vi "系统设置.vi"() -> ()   [LabVIEW 2016]
uses:
  <vilib>/Utility/miscctls.llb/LVPointTypeDef.ctl
  <vilib>/Utility/config.llb/Read Key (U32).vi
  <vilib>/Utility/config.llb/Write Key (I32).vi
  <vilib>/ptbypt/NI_PtbyPt.lvlib
  PLC/PLC.lvlib
  <vilib>/Utility/config.llb/NI_LVConfig.lvlib
panel:
  in  "24H周期设置":T1(xcontrol)
  in  "采水模式":enum16{"使用采水泵", "不使用采水泵"}(ring)
  in  "运行模式":enum16{"维护模式", "常规模式", "应急模式", "质控模式"}(ring)
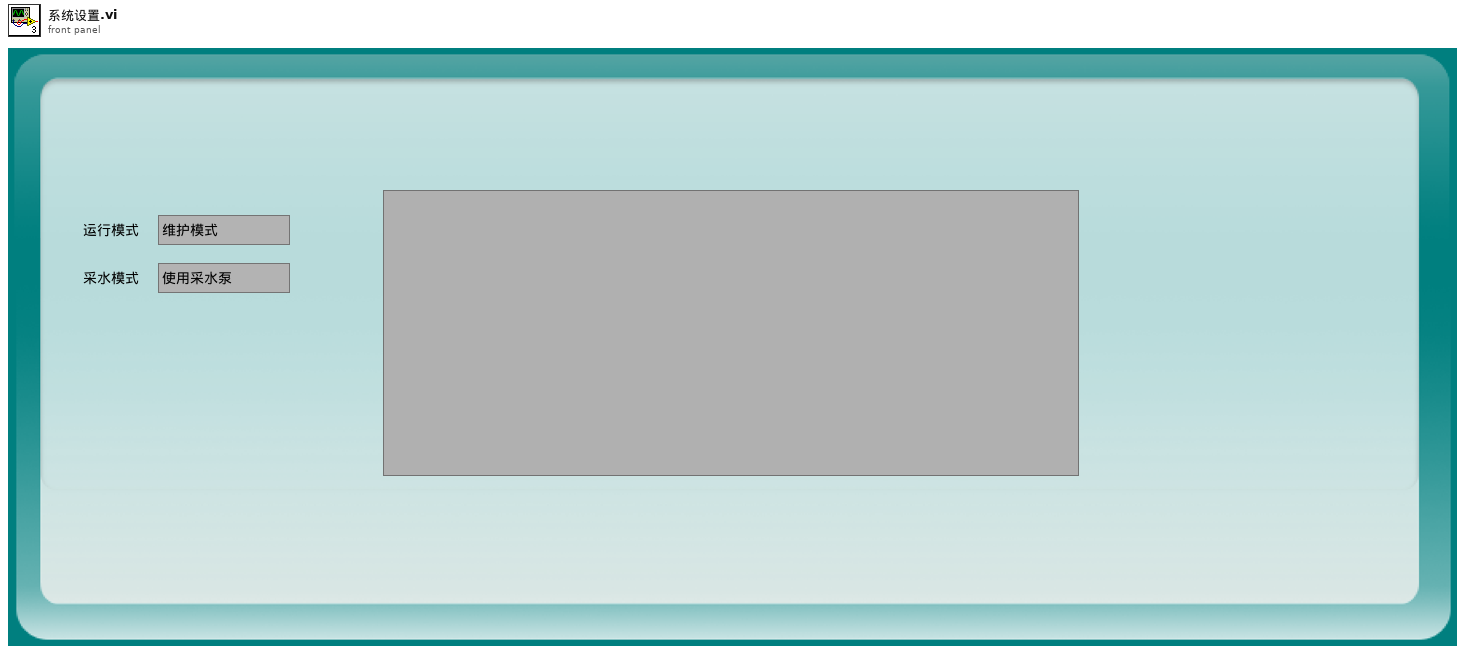
[diagram p1: front panel]
types:
  T1 = cluster{"00H":bool, "01H":bool, "02H":bool, "03H":bool, "04H":bool, "05H":bool, "06H":bool, "07H":bool, "08H":bool, "09H":bool, "10H":bool, "11H":bool, "12H":bool, "13H":bool, "14H":bool, "15H":bool, "16H":bool, "17H":bool, "18H":bool, "19H":bool, "20H":bool, "21H":bool, "22H":bool, "23H":bool}
  T2 = typedef "LVPointTypeDef.ctl" = cluster{"Horizontal":i16, "Vertical":i16}
  T3 = typedef "NI_LVConfig.lvlib/Config Data RefNum.ctl" = refnum<k1>
  T4 = cluster{"是否启用仪器":bool, "CODMn":cluster{"启动测量模式":cluster{"测量模式":enum16{"水样测量", "标样核查", "零点核查", "加标回收", "平行样", "校零", "校标"}}, "确定按钮":bool}, "采水模式":enum16{"使用采水泵", "不使用采水泵"}}
  T5 = enum16{"水样测量", "标样核查", "零点核查", "加标回收", "平行样", "校零", "校标"}
  T6 = cluster{"运行模式":enum16{"维护模式", "常规模式", "应急模式", "质控模式"}}
  T7 = typedef "LVDateTimeRec.ctl" = cluster{"秒数的小数部分":dbl, "秒":i32, "分":i32, "时":i32, "日":i32, "月":i32, "年":i32, "天数（周）":i32, "天数（年）":i32, "DST":i32}
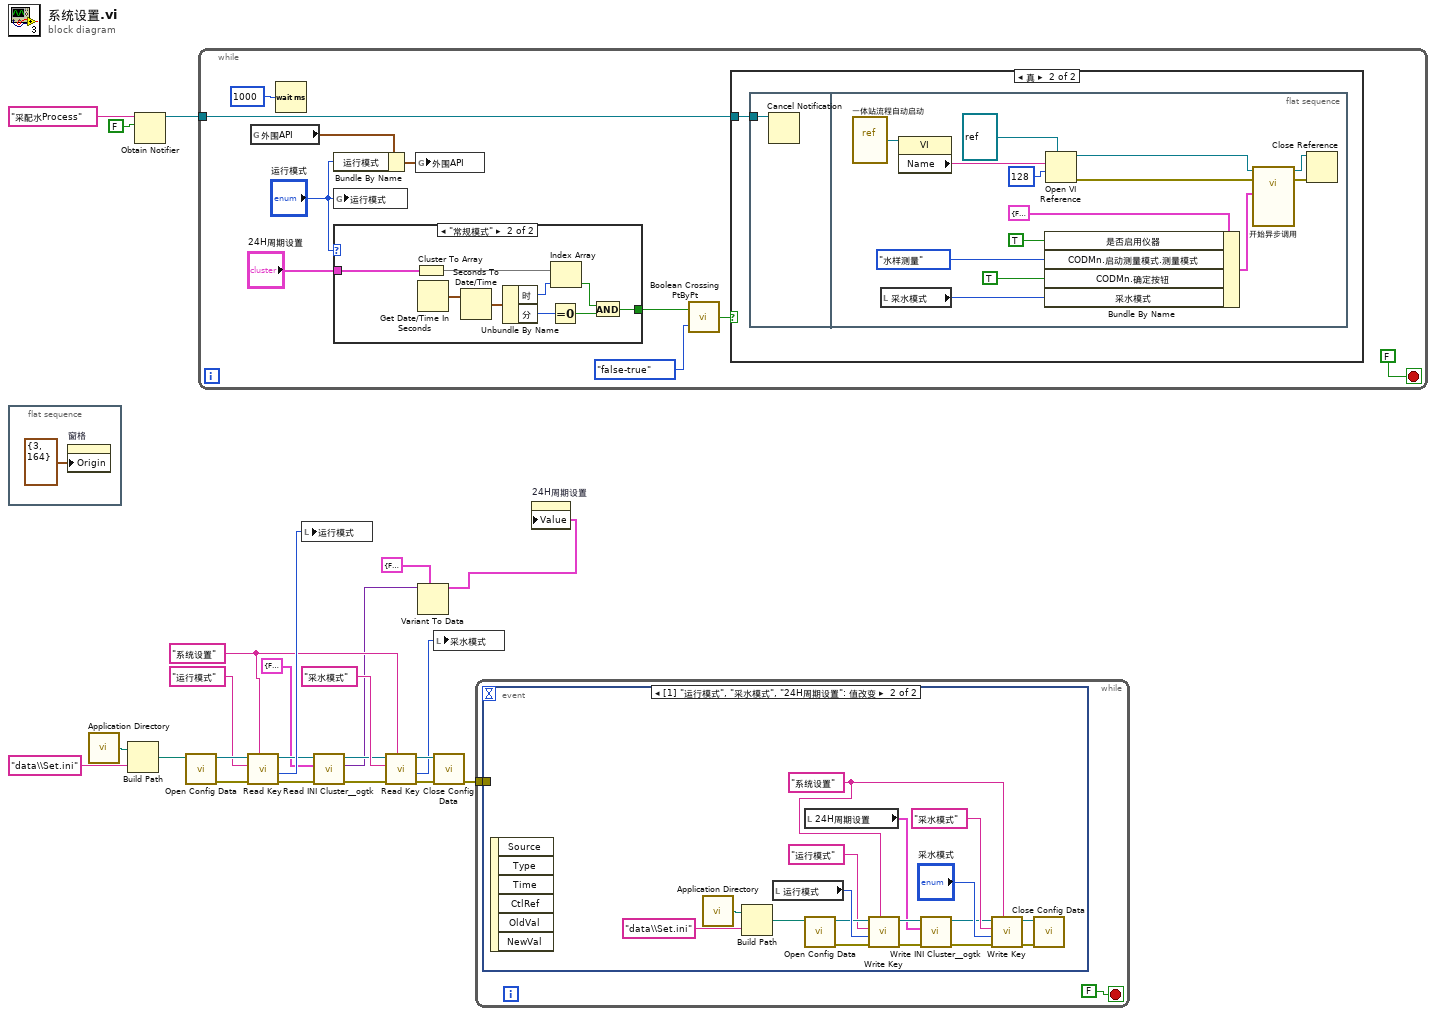
[diagram p0: block diagram]
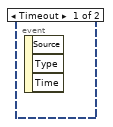
[diagram p4: hidden frame]
diagram:
  w9 = "系统设置" ("section")
  n1 = flat-sequence {
    frame #0 {
      n2 = property on="窗格" class="Pane"("Origin"=T2 {"Horizontal"=3, "Vertical"=164} ("原点")) -> ()  [unwired: 2 in, 2 out]
    }
  }
  n3 = call <vilib>:"Application Directory.vi"() -> ("Application Directory"=w19:path)
  n4 = Build Path(base path=w19, name or relative path="data\\Set.ini" ("名称或相对路径")) -> (appended path=w17:path)
  n5 = Obtain Notifier(name (unnamed)="采配水Process" ("名称（未命名）"), notification data type=FALSE) -> (notifier out=w22:refnum<notifier>)  [unwired: 2 in, 2 out]
  n6 = call <vilib>:"Open Config Data.vi"("configuration file path"=w17) -> ("error out"=w20:errorcluster, "refnum"=w21:T3)  [unwired: 8 in, 1 out]
  n7 = while {
    tunnel: w22 -> [w33]
    stop <- FALSE stop-if-true
    n8 = global read "VAR总磷氨氮全局变量.vi" "外围API"() -> (w28:T6)
    n9 = Wait (ms)(milliseconds to wait=u32 1000 ("等待时间（毫秒）")) -> ()  [unwired: 1 out]
    n10 = Bundle By Name(cluster=w28, "运行模式"="运行模式") -> (w27:T6)
    n11 = global write "系统变量.vi" "运行模式"("运行模式") -> ()
    n12 = case shown="\"常规模式\"" "运行模式" {
      tunnel: [_ w56] -> w32
      tunnel: "24H周期设置" -> [_ w55]
      frame "维护模式", Default {
      }
      frame "常规模式" {
        n13 = Cluster To Array(cluster=w55) -> (array=w54:bool[])
        n14 = Get Date/Time In Seconds() -> (seconds since 1Jan1904=w60:timestamp)
        n15 = Seconds To Date/Time(time stamp (now)=w60) -> (date time rec=w59:T7)  [unwired: 1 in]
        n16 = Unbundle By Name(w59) -> ("时"=w53:i32, "分"=w58:i32)
        n17 = Equal To 0?(x=w58) -> (x = 0?=w57:bool)
        n18 = Index Array(array=w54, index=w53) -> (element=w52:bool)
        n19 = And(x=w52, y=w57) -> (x .and. y?=w56:bool)
      }
    }
    n20 = global write "VAR总磷氨氮全局变量.vi" "外围API"(w27) -> ()
    n21 = call <vilib>:"Boolean Crossing PtByPt.vi"("direction"=enum16{"either", "false-true", "true-false"}."false-true", "input"=w32) -> ("crossing"=w30:bool)  [unwired: 1 in]
    n22 = case shown="真" w30 {
      tunnel: w33 -> [_ w36]
      frame False {
      }
      frame True {
        n23 = flat-sequence {
          tunnel: w36 -> [w37]
          frame #0 {
            n24 = Cancel Notification(0:w37) -> ()  [unwired: 1 in, 3 out]
          }
          frame #1 {
            n25 = vi-ref "一体站流程自动启动.vi"() -> (w51:refnum<vi>)
            n26 = local read "采水模式"() -> (w39:enum16{"使用采水泵", "不使用采水泵"})
            n27 = property class="VI"(reference=w51) -> ("Name"=w50:string)  [unwired: 1 in, 2 out]
            n28 = Bundle By Name(cluster=T4 {"是否启用仪器"=FALSE, "CODMn"={"启动测量模式"={"测量模式"=enum."水样测量"}, "确定按钮"=FALSE}, "采水模式"=enum."使用采水泵"} ("参数"), "是否启用仪器"=TRUE, "CODMn.启动测量模式.测量模式"=T5."水样测量", "CODMn.确定按钮"=TRUE, "采水模式"=w39) -> (w38:T4)
            n29 = Open VI Reference(type specifier VI Refnum (for type only)=refnum<vi> refnum, vi path=w50, options=128 ("选项")) -> (vi reference=w48:refnum<vi>, error out=w45:errorcluster)  [unwired: 3 in]
            n30 = call-by-ref "开始异步调用"(reference=w48, error in=w45, "参数"=w38) -> (reference out=w46:refnum<vi>, error out=w44:errorcluster)  [unwired: 11 in]
            n31 = Close Reference(reference=w46, error in (no error)=w44) -> ()  [unwired: 1 out]
          }
        }
      }
    }
  }
  n32 = call-poly <vilib>:"Read Key.vi"("section"=w9, "error in (no error)"=w20, "key"="运行模式" ("section"), "refnum"=w21) -> ("error out"=w6:errorcluster, "value"=w16:u32, "refnum out"=w8:T3)  [unwired: 4 in, 1 out]
  n33 = local write "运行模式"(w16) -> ()
  n34 = call <userlib>:"Read INI Cluster__ogtk.vi"("error in (no error)"=w6, "INI Fomatted Cluster Type"=T1 {"00H"=FALSE, "01H"=FALSE, "02H"=FALSE, "03H"=FALSE, "04H"=FALSE, "05H"=FALSE, "06H"=FALSE, "07H"=FALSE, "08H"=FALSE, "09H"=FALSE, "10H"=FALSE, "11H"=FALSE, "12H"=FALSE, "13H"=FALSE, "14H"=FALSE, "15H"=FALSE, "16H"=FALSE, "17H"=FALSE, "18H"=FALSE, "19H"=FALSE, "20H"=FALSE, "21H"=FALSE, "22H"=FALSE, "23H"=FALSE} ("24H周期设置"), "refnum"=w8) -> ("error out"=w5:errorcluster, "INI Fomatted Cluster"=w4:variant, "dup refnum"=w7:T3)  [unwired: 4 in, 2 out]
  n35 = call-poly <vilib>:"Read Key.vi"("section"=w9, "error in (no error)"=w5, "key"="采水模式", "refnum"=w7) -> ("error out"=w12:errorcluster, "value"=w10:u32, "refnum out"=w13:T3)  [unwired: 4 in, 1 out]
  n36 = Variant To Data(type=T1 {"00H"=FALSE, "01H"=FALSE, "02H"=FALSE, "03H"=FALSE, "04H"=FALSE, "05H"=FALSE, "06H"=FALSE, "07H"=FALSE, "08H"=FALSE, "09H"=FALSE, "10H"=FALSE, "11H"=FALSE, "12H"=FALSE, "13H"=FALSE, "14H"=FALSE, "15H"=FALSE, "16H"=FALSE, "17H"=FALSE, "18H"=FALSE, "19H"=FALSE, "20H"=FALSE, "21H"=FALSE, "22H"=FALSE, "23H"=FALSE} ("24H周期设置"), Variant=w4) -> (data=w1:T1)  [unwired: 1 in, 1 out]
  n37 = local write "采水模式"(w10) -> ()
  n38 = call <vilib>:"Close Config Data.vi"("error in (no error)"=w12, "refnum"=w13) -> ("error out"=w14:errorcluster)  [unwired: 8 in, 1 out]
  n39 = while {
    tunnel: w14 -> [w61]
    stop <- FALSE stop-if-true
    n40 = event shown="[1] \"运行模式\", \"采水模式\", \"24H周期设置\": 值改变" {
      selector: _ -> [_ _]
      dyn-events: _ -> [_ _]
      timeout: _ -> [_ _]
      tunnel: w61 -> [_ _]
      event Timeout {
        n41 = event-data() -> ()  [unwired: 1 in, 3 out]
      }
      event "运行模式", "采水模式", "24H周期设置": Value Change {
        w68 = "系统设置" ("section")
        n42 = event-data() -> ()  [unwired: 1 in, 6 out]
        n43 = call <vilib>:"Application Directory.vi"() -> ("Application Directory"=w76:path)
        n44 = Build Path(base path=w76, name or relative path="data\\Set.ini" ("名称或相对路径")) -> (appended path=w74:path)
        n45 = local read "运行模式"() -> (w79:enum16{"维护模式", "常规模式", "应急模式", "质控模式"})
        n46 = local read "24H周期设置"() -> (w63:T1)
        n47 = call <vilib>:"Open Config Data.vi"("configuration file path"=w74) -> ("error out"=w77:errorcluster, "refnum"=w78:T3)  [unwired: 8 in, 1 out]
        n48 = call-poly <vilib>:"Write Key.vi"("section"=w68, "error in (no error)"=w77, "value"=w79, "key"="运行模式" ("section"), "refnum"=w78) -> ("error out"=w66:errorcluster, "refnum out"=w67:T3)  [unwired: 4 in, 1 out]
        n49 = call <userlib>:"Write INI Cluster__ogtk.vi"("error in (no error)"=w66, "INI Fomatted Cluster"=w63, "refnum"=w67) -> ("error out"=w64:errorcluster, "dup refnum"=w65:T3)  [unwired: 7 in]
        n50 = call-poly <vilib>:"Write Key.vi"("section"=w68, "error in (no error)"=w64, "value"="采水模式", "key"="采水模式", "refnum"=w65) -> ("error out"=w69:errorcluster, "refnum out"=w70:T3)  [unwired: 4 in, 1 out]
        n51 = call <vilib>:"Close Config Data.vi"("error in (no error)"=w69, "refnum"=w70) -> ()  [unwired: 8 in, 2 out]
      }
    }
  }
  n52 = property on="24H周期设置" class="24H周期设置 (严格)"("Value"=w1) -> ()  [unwired: 2 in, 2 out]
